vi "record P0(air) format.vi"(9 "wave length":dbl[](array[numeric]), 10 "P0(air)":dbl[](array[numeric]), 11 "number":i32) -> (3 "P0(air) data":string[][](array[string]))   [LabVIEW 2020]
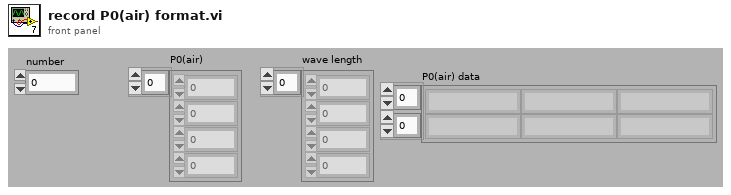
[diagram p1: front panel]
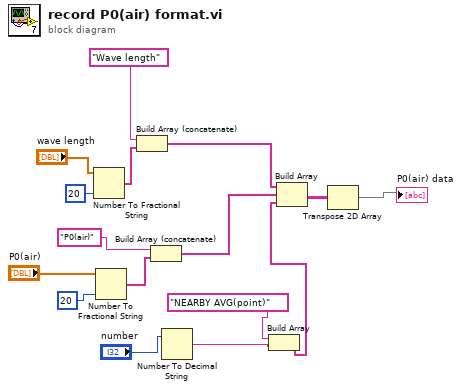
[diagram p0: block diagram]
diagram:
  n1 = Number To Fractional String(number="wave length", precision (6)=i16 20) -> (F-format string=w14:string[])  [unwired: 2 out]
  n2 = Number To Fractional String(number="P0(air)", precision (6)=i16 20) -> (F-format string=w11:string[])  [unwired: 2 out]
  n3 = Build Array (concatenate)("Wave length" ("Numeric"), w14) -> (w8:string[])
  n4 = Build Array (concatenate)("P0(air)" ("Numeric"), w11) -> (w7:string[])
  n5 = Number To Decimal String(number="number") -> (decimal integer string=w5:string)  [unwired: 1 out]
  n6 = Build Array("NEARBY AVG(point)" ("Numeric"), w5) -> (w4:string[])
  n7 = Build Array(w8, w7, w4) -> (w3:string[][])
  n8 = Transpose 2D Array(2D array=w3) -> (transposed array=→"P0(air) data":string[][])
